vi "CmdHandler.vi"(10 "Message":T1={"update_id"=0, "from"="", "text"="", "date"=timestamp(2082844800 s since 1904-01-01), "chat_id"=0, "type"="", "reply_to_message.text"="", "message_id"=0}, 11 "GlobalDataRef":refnum<data-value>) -> (0 "Error":errorcluster)   [LabVIEW 2015]
uses:
  Telegram/Methods/TypeDefs/Message.ctl
  ProjectFiles/TypeDefs/GlobalData.ctl
  Telegram/Methods/TypeDefs/ReplyKeyboardMarkup.ctl
  ProjectFiles/TypeDefs/StatusLogMessages.ctl
  Telegram/Methods/TypeDefs/SendMessageType.ctl
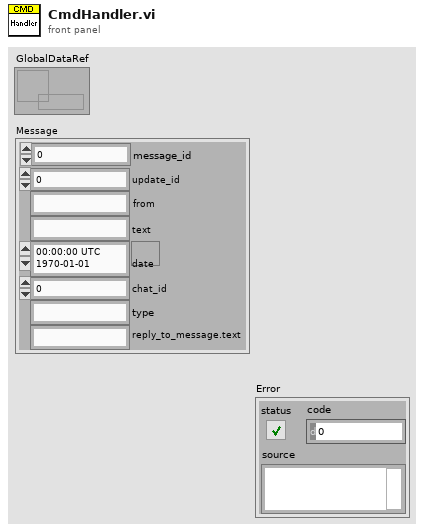
[diagram p1: front panel]
types:
  T1 = typedef "Message.ctl" = cluster{"update_id":u32, "from":string, "text":string, "date":timestamp, "chat_id":i32, "type":string, "reply_to_message.text":string, "message_id":u32}
  T2 = typedef "CommandList.ctl" = string[]
  T3 = cluster{"Cmd":T2, "Param":string[], "CmdText":string, "ChatId":i32}
  T4 = typedef "SendMessageType.ctl" = enum16{"Text", "ReplyKeyboardMarkup", "ReplyKeyboardRemove"}
  T5 = typedef "StatusLogMessages.ctl" = string
  T6 = cluster{"Period":u32, "DutyCycle":u32, "LED#":string}
  T7 = typedef "ReplyKeyboardMarkup.ctl" = cluster{"keyboard":cluster{"text":string, "req_loc":bool}[][], "resize_keyboard":bool, "one_time_keyboard":bool, "selective":bool}
  T8 = cluster{"Period":u32, "DutyCycle":u32, "Cmd":string}
  T9 = typedef "GlobalData.ctl" = cluster{"FPGA VI Ref":refnum<k20>, "Token":string, "ActiveChats":cluster{"ChatId":i32, "Type":string}[], "ActiveKeyboards":cluster{"Chat#":i32, "ReplyKeyboardMarkup":T7}[], "RefStringIn":refnum<vi>}
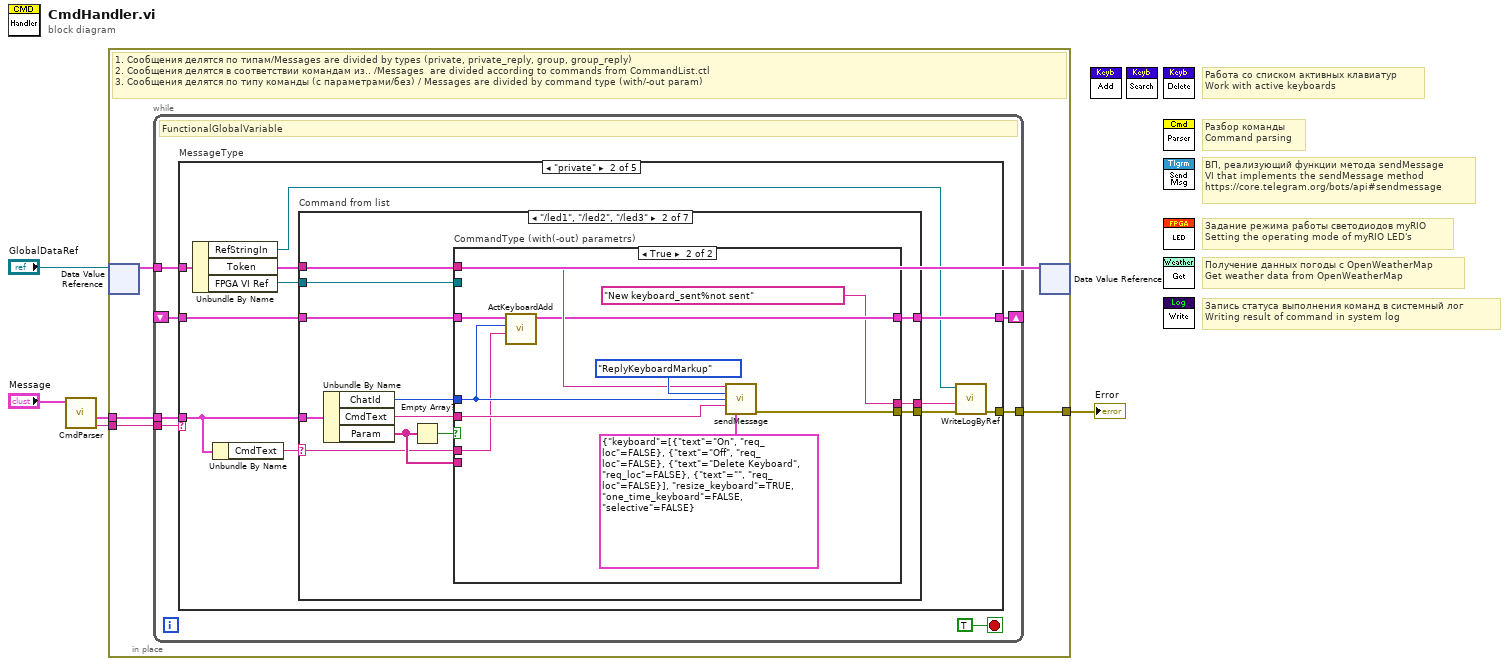
[diagram p0: block diagram]
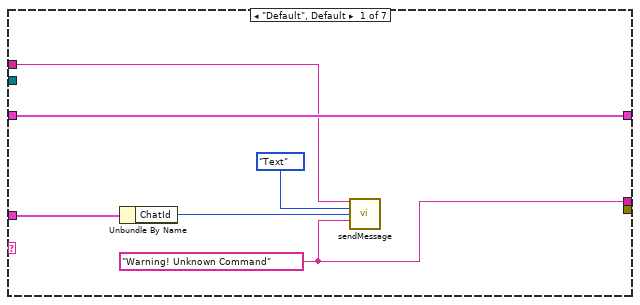
[diagram p3: hidden frame]
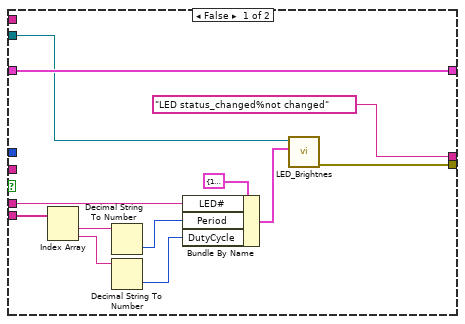
[diagram p4: hidden frame]
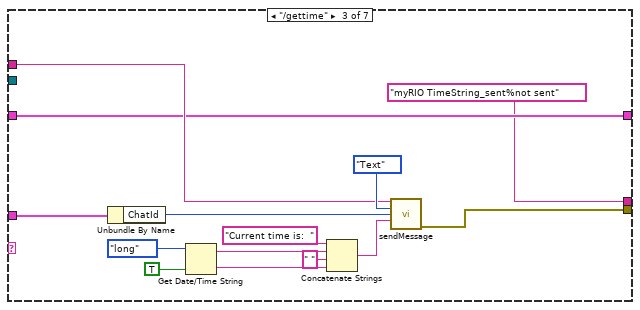
[diagram p5: hidden frame]
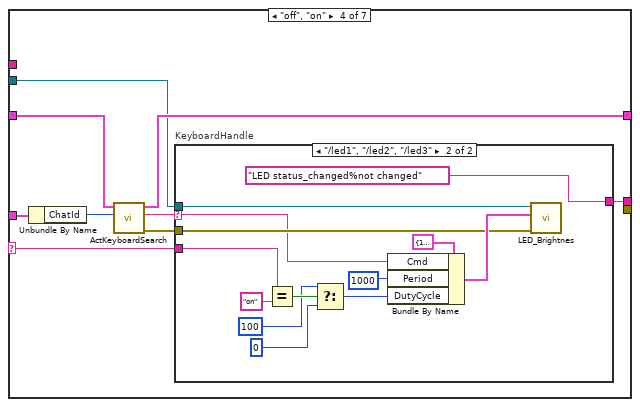
[diagram p6: hidden frame]
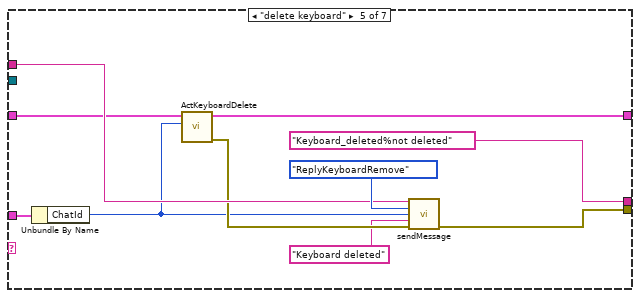
[diagram p8: hidden frame]
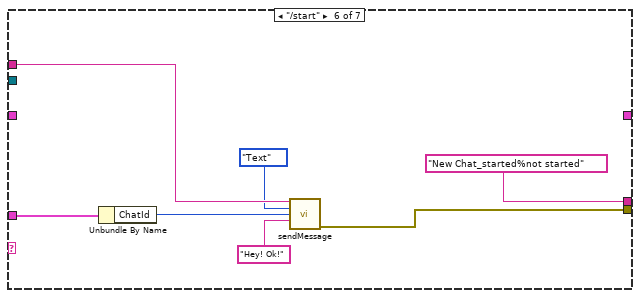
[diagram p9: hidden frame]
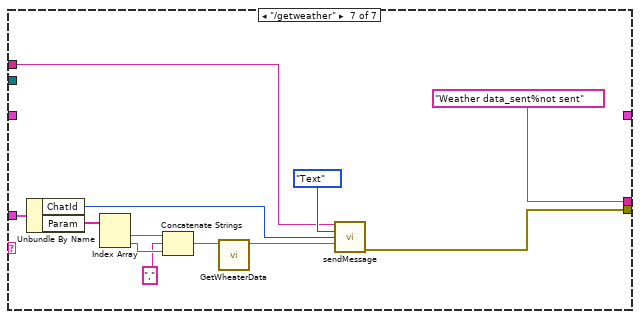
[diagram p10: hidden frame]
diagram:
  # "Запись статуса выполнения команд в системный лог\nWriting result of command in system log"
  # "Получение данных погоды с OpenWeatherMap\nGet weather data from OpenWeatherMap"
  # "Задание режима работы светодиодов myRIO\nSetting the operating mode of myRIO LED's"
  # "ВП, реализующий функции метода sendMessage\nVI that implements the sendMessage method\nhttps://core.telegram.org/bots/api#sendmessage"
  # "Разбор команды\nCommand parsing"
  # "Работа со списком активных клавиатур\nWork with active keyboards"
  n1 = call "CmdParser.vi"("message"="Message") -> ("msg_type"=w3:string, "Cmd"=w4:T3)  [unwired: 7 in, 2 out]
  n2 = in-place {
    in-place-border: w4 -> [w9]
    in-place-border: w3 -> [w8]
    in-place-border: [w7] -> w2
    # "1. Сообщения делятся по типам/Messages are divided by types (private, private_reply, group, group_reply)\n2. Сообщения делятся в соответствии командам из.. /Messages  are divided according to commands from CommandList.ctl\n3. Сообщения делятся по типу команды (с параметрами/без) / Messages are divided by command type (with/-out param)"
    n3 = in-place-dvr #1("GlobalDataRef") -> (w6:T9)  [unwired: 1 out]
    n4 = while {
      tunnel: w6 -> [w10]
      tunnel: w9 -> [w14]
      tunnel: w8 -> [w15]
      tunnel: [w13] -> w7
      shift-right: [w12] -> _
      shift-left: _ -> [w11]
      stop <- TRUE stop-if-true
      # "FunctionalGlobalVariable"
      n5 = case "MessageType" shown="\"private\"" w15 {
        tunnel: w10 -> [_ w27 _ _ _]
        tunnel: w14 -> [_ w25 _ _ _]
        tunnel: [_ w21 _ _ _] -> w13
        tunnel: [w17 w24 w134 w135 w136] -> w12
        tunnel: w11 -> [w17 w23 w134 w135 w136]
        frame Default {
        }
        frame "private" {
          n6 = Unbundle By Name(w27) -> ("RefStringIn"=w19:refnum<vi>, "Token"=w26:string, "FPGA VI Ref"=w18:refnum<k20>)
          n7 = Unbundle By Name(w25) -> ("CmdText"=w28:string)
          n8 = case "Command from list" shown="\"/led1\", \"/led2\", \"/led3\"" w28 {
            selector: w28 -> [_ w40 _ w86 _ _ _]
            tunnel: w26 -> [w31 w42 w71 _ w113 w120 w125]
            tunnel: w25 -> [w33 w46 w74 w89 w112 w121 w133]
            tunnel: [_ w36 w72 _ w111 w118 w126] -> w22
            tunnel: [w34 w39 w70 w90 w109 _ _] -> w24
            tunnel: w23 -> [w34 w38 w70 w91 w110 _ _]
            tunnel: w18 -> [_ w37 _ w85 _ _ _]
            tunnel: [w29 w35 T5 "myRIO TimeString_sent%not sent" ("MessagesList") w84 T5 "Keyboard_deleted%not deleted" ("MessagesList") T5 "New Chat_started%not started" ("MessagesList") T5 "Weather data_sent%not sent" ("MessagesList")] -> w20
            frame "Default", Default {
              w29 = T5 "Warning! Unknown Command" ("MessagesList")
              n9 = Unbundle By Name(w33) -> ("ChatId"=w32:i32)
              n10 = call "sendMessage.vi"("Token"=w31, "MsgType"=SendMessageType."Text", "ChatId"=w32, "Text"=w29) -> ()  [unwired: 11 in, 1 out]
            }
            frame "/led1", "/led2", "/led3" {
              n11 = Unbundle By Name(w46) -> ("ChatId"=w44:i32, "CmdText"=w43:string, "Param"=w41:string[])
              n12 = Empty Array?(array=w41) -> (empty?=w45:bool)
              n13 = case "CommandType (with(-out) parametrs)" shown="True" w45 {
                tunnel: w44 -> [_ w63]
                tunnel: w43 -> [_ w66]
                tunnel: w42 -> [_ w67]
                tunnel: [w50 w60] -> w36
                tunnel: w41 -> [w54 _]
                tunnel: w40 -> [w53 w62]
                tunnel: [w52 w64] -> w39
                tunnel: w38 -> [w52 w65]
                tunnel: w37 -> [w51 _]
                tunnel: [T5 "LED status_changed%not changed" ("MessagesList") T5 "New keyboard_sent%not sent" ("MessagesList")] -> w35
                frame False {
                  n14 = Index Array(array=w54) -> (element #1=w55:string, element #2=w56:string)  [unwired: 2 in]
                  n15 = Decimal String To Number(string=w55) -> (number=w57:i32)  [unwired: 2 in, 1 out]
                  n16 = Decimal String To Number(string=w56) -> (number=w58:i32)  [unwired: 2 in, 1 out]
                  n17 = Bundle By Name(cluster=T6 {"Period"=1000, "DutyCycle"=0, "LED#"="/led1"} ("LEDParam"), "LED#"=w53, "Period"=w57, "DutyCycle"=w58) -> (w48:T6)
                  n18 = call "LED_Brightnes.vi"("LEDParam"=w48, "FPGA VI"=w51) -> ("error out"=w50:errorcluster)  [unwired: 8 in, 1 out]
                }
                frame True {
                  n19 = call "ActKeyboardAdd.vi"("Cmd"=w62, "ChatId"=w63, "ActKeyboards in"=w65) -> ("ActKeyboards out"=w64:cluster{"ChatId":i32, "Cmd":string}[])  [unwired: 7 in, 1 out]
                  n20 = call "sendMessage.vi"("Token"=w67, "MsgType"=SendMessageType."ReplyKeyboardMarkup", "ChatId"=w63, "Text"=w66, "ReplyKeyboardMarkup"=T7 {"keyboard"=[[{"text"="On", "req_loc"=FALSE}, {"text"="Off", "req_loc"=FALSE}], [{"text"="Delete Keyboard", "req_loc"=FALSE}, {"text"="", "req_loc"=FALSE}]], "resize_keyboard"=TRUE, "one_time_keyboard"=FALSE, "selective"=FALSE}) -> ("error out"=w60:errorcluster)  [unwired: 10 in]
                }
              }
            }
            frame "/gettime" {
              n21 = Unbundle By Name(w74) -> ("ChatId"=w73:i32)
              n22 = Get Date/Time String(date format (0)=enum16{"short", "long", "abbreviated"}."long", want seconds? (F)=TRUE) -> (date string=w79:string, time string=w80:string)  [unwired: 1 in]
              n23 = Concatenate Strings("Current time is:  " ("string"), w79, " " ("string"), w80) -> (w76:string)
              n24 = call "sendMessage.vi"("Token"=w71, "MsgType"=SendMessageType."Text", "ChatId"=w73, "Text"=w76) -> ("error out"=w72:errorcluster)  [unwired: 11 in]
            }
            frame "off", "on" {
              n25 = Unbundle By Name(w89) -> ("ChatId"=w88:i32)
              n26 = call "ActKeyboardSearch.vi"("ChatId"=w88, "ActKeyboards in"=w91) -> ("Error"=w87:errorcluster, "Cmd"=w83:string, "ActKeyboards out"=w90:cluster{"ChatId":i32, "Cmd":string}[])  [unwired: 6 in, 1 out]
              n27 = case "KeyboardHandle" shown="\"/led1\", \"/led2\", \"/led3\"" w83 {
                selector: w83 -> [_ w94]
                tunnel: w87 -> [_ w98]
                tunnel: w86 -> [_ w97]
                tunnel: w85 -> [_ w96]
                tunnel: [_ T5 "LED status_changed%not changed" ("MessagesList")] -> w84
                frame "Default", Default {
                }
                frame "/led1", "/led2", "/led3" {
                  n28 = Equal?(x=w97, y="on") -> (x = y?=w102:bool)
                  n29 = Select(t=u32 100 ("upper limit"), s=w102, f=u32 0 ("lower limit")) -> (s? t:f=w101:u32)
                  n30 = Bundle By Name(cluster=T8 {"Period"=1000, "DutyCycle"=0, "Cmd"="/led1"} ("LEDParam"), "Cmd"=w94, "Period"=u32 1000, "DutyCycle"=w101) -> (w103:T8)
                  n31 = call "LED_Brightnes.vi"("error in (no error)"=w98, "LEDParam"=w103, "FPGA VI"=w96) -> ()  [unwired: 7 in, 2 out]
                }
              }
            }
            frame "delete keyboard" {
              n32 = Unbundle By Name(w112) -> ("ChatId"=w106:i32)
              n33 = call "ActKeyboardDelete.vi"("ChatId"=w106, "ActKeyboards in"=w110) -> ("Error"=w107:errorcluster, "ActKeyboards out"=w109:cluster{"ChatId":i32, "Cmd":string}[])  [unwired: 8 in]
              n34 = call "sendMessage.vi"("Token"=w113, "MsgType"=SendMessageType."ReplyKeyboardRemove", "ChatId"=w106, "Text"="Keyboard deleted", "error in"=w107) -> ("error out"=w111:errorcluster)  [unwired: 10 in]
            }
            frame "/start" {
              n35 = Unbundle By Name(w121) -> ("ChatId"=w119:i32)
              n36 = call "sendMessage.vi"("Token"=w120, "MsgType"=SendMessageType."Text", "ChatId"=w119, "Text"="Hey! Ok!") -> ("error out"=w118:errorcluster)  [unwired: 11 in]
            }
            frame "/getweather" {
              n37 = Unbundle By Name(w133) -> ("ChatId"=w124:i32, "Param"=w132:string[])
              n38 = Index Array(array=w132) -> (element #1=w131:string, element #2=w130:string)  [unwired: 2 in]
              n39 = Concatenate Strings(w131, "," ("string"), w130) -> (w128:string)
              n40 = call "GetWheaterData.vi"("Locaion"=w128) -> ("WeatherString"=w123:string)  [unwired: 10 in]
              n41 = call "sendMessage.vi"("Token"=w125, "MsgType"=SendMessageType."Text", "ChatId"=w124, "Text"=w123) -> ("error out"=w126:errorcluster)  [unwired: 11 in]
            }
          }
          n42 = call "WriteLogByRef.vi"("ErrorIn"=w22, "MessagesList"=w20, "RefStringIn"=w19) -> ("ErrorOut"=w21:errorcluster)  [unwired: 7 in, 1 out]
        }
        frame "private_reply" {
        }
        frame "group" {
        }
        frame "group_reply" {
        }
      }
    }
    n43 = in-place-dvr #1(w6) -> ()  [unwired: 2 out]
  }
  "Error" <- w2
